vi "BMark_Get Bookmarks for VI.vi"(0 "VI":T2, 1 "App Infos In":T3[](array[typedef]), 7 "VI Cache In":T2[](array[typedef]), 9 "Bookmark Cache In":cluster{"BookmarkInfo":T1}[](array[cluster]), 11 "Error In":errorcluster, 12 "App Cache In":refnum<vi>[](array[refnum])) -> (3 "App Infos Out":T3[](array[typedef]), 4 "Bookmarks":T4, 6 "Possible Undisplayed Bookmarks":bool, 8 "VI Cache Out":T2[](array[typedef]), 10 "Bookmark Cache Out":cluster{"BookmarkInfo":T1}[](array[cluster]), 14 "App Cache Out":refnum<vi>[](array[refnum]), 15 "Error Out":errorcluster)   [LabVIEW 2018, in "Bookmark Manager.lvlib"]
uses:
  Bookmark Manager.lvlib
  Controls/BMark_VI_Identifier.ctl
  <vilib>/addons/analyzer/_analyzerctrls.llb/VIAnCtl Analysis App Info.ctl
  Controls/BMark_Array of Bookmarks.ctl
  Controls/BMark_Bookmark Cluster.ctl
  <vilib>/Utility/miscctls.llb/LVBookmarkInfoTypeDef.ctl
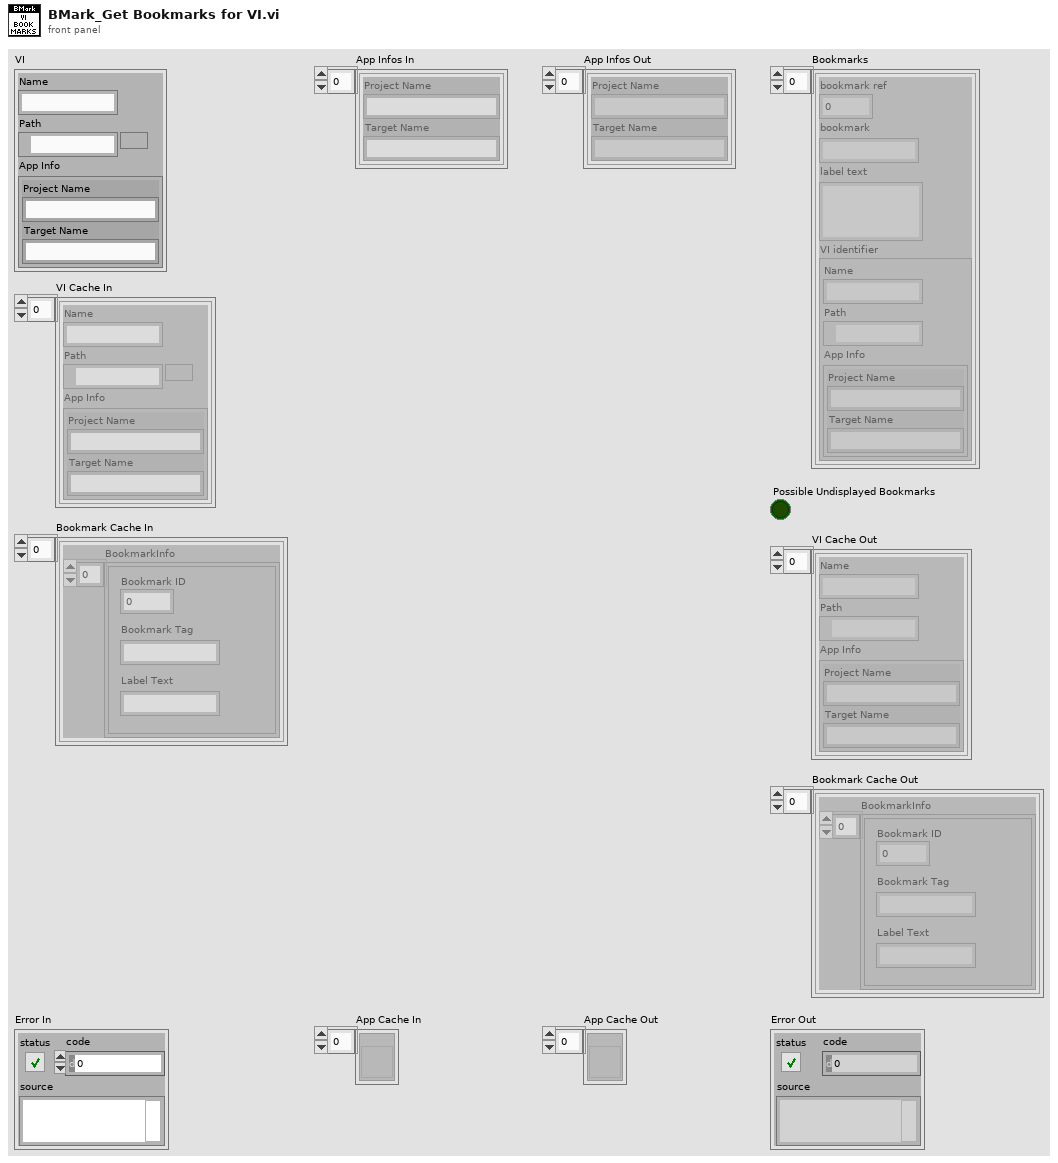
[diagram p1: front panel]
types:
  T1 = typedef "LVBookmarkInfoTypeDef.ctl" = cluster{"Bookmark ID":u32, "Bookmark Tag":string, "Label Text":string}[]
  T2 = typedef "Bookmark Manager.lvlib/BMark_VI_Identifier.ctl" = cluster{"Name":string, "Path":path, "App Info":T3}
  T3 = typedef "VIAnCtl Analysis App Info.ctl" = cluster{"Project Name":string, "Target Name":string}
  T4 = typedef "Bookmark Manager.lvlib/BMark_Array of Bookmarks.ctl" = T5[]
  T5 = typedef "Bookmark Manager.lvlib/BMark_Bookmark Cluster.ctl" = cluster{"bookmark ref":i32, "bookmark":string, "label text":string, "VI identifier":T2}
  T6 = cluster{"Bookmark Reference":u32, "Bookmark Tag":string, "Label Text":string, "VI":T2}
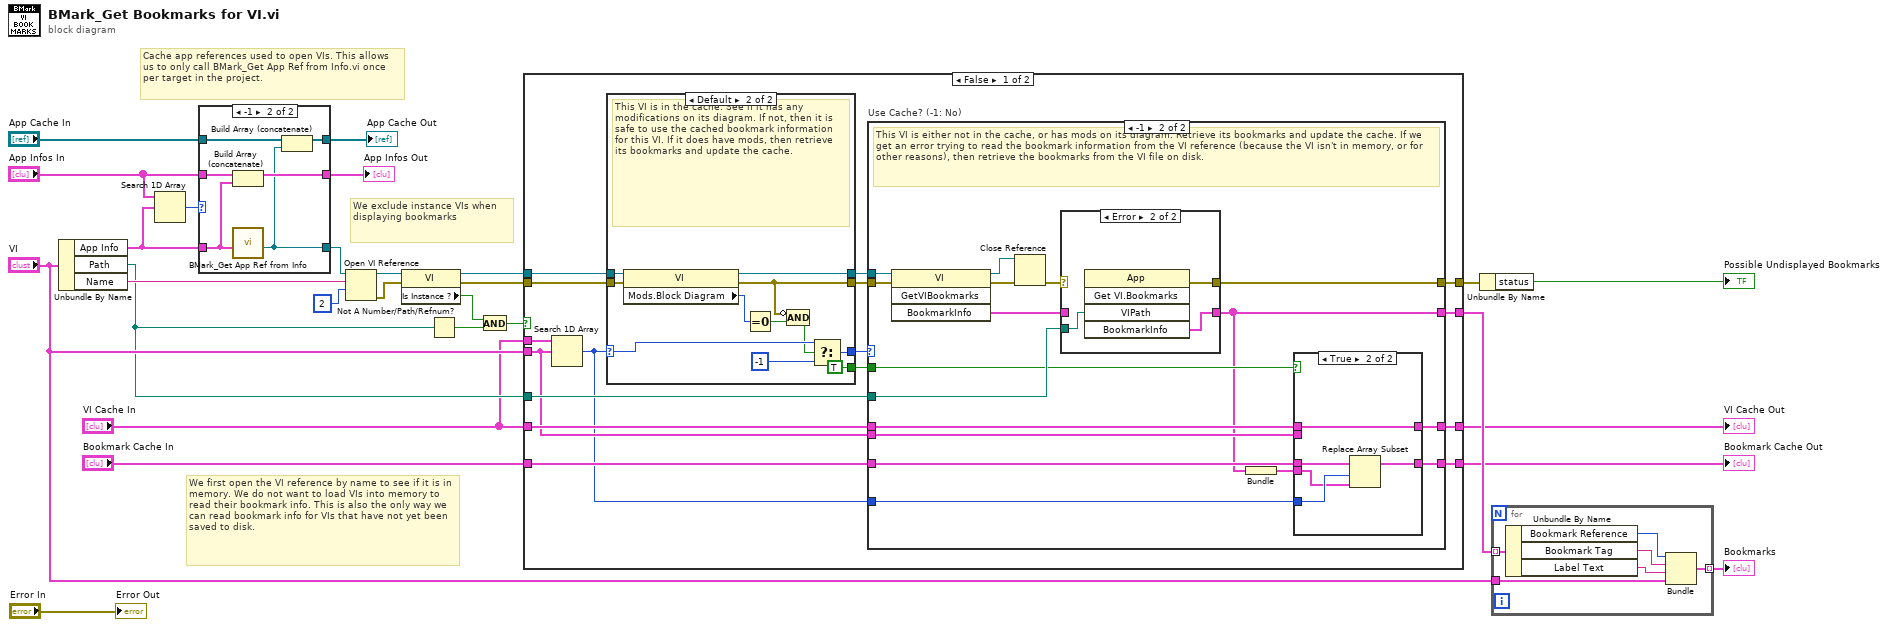
[diagram p0: block diagram]
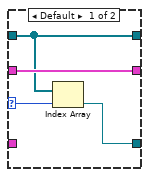
[diagram p2: hidden frame]
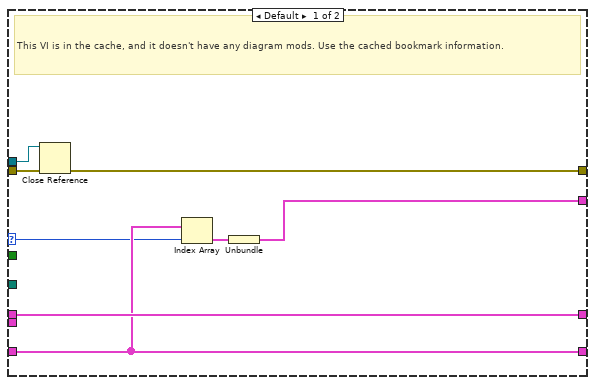
[diagram p4: hidden frame]
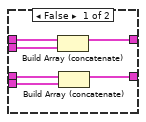
[diagram p5: hidden frame]
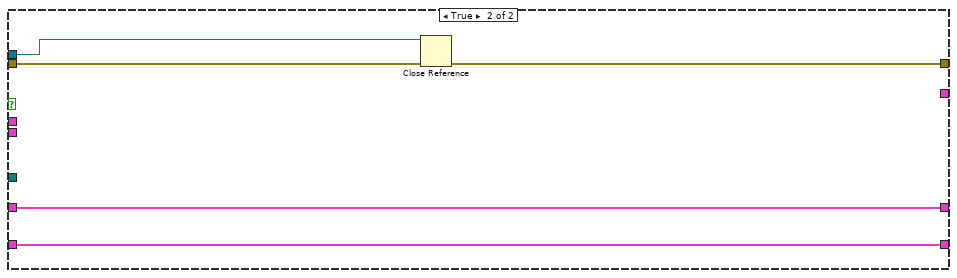
[diagram p7: hidden frame]
diagram:
  # "Cache app references used to open VIs. This allows us to only call BMark_Get App Ref from Info.vi once per target in the project."
  # "We exclude instance VIs when displaying bookmarks"
  # "We first open the VI reference by name to see if it is in memory. We do not want to load VIs into memory to read their bookmark info. This is also the only way we can read bookmark info for VIs that have not yet been saved to disk."
  n1 = Unbundle By Name("VI") -> ("App Info"=w16:T3, "Path"=w6:path, "Name"=w25:string)
  n2 = Search 1D Array(1D array="App Infos In", element=w16) -> (index of element=w15:i32)  [unwired: 1 in]
  n3 = case shown="-1" w15 {
    selector: w15 -> [w31 _]
    tunnel: [w29 w32] -> w24
    tunnel: w16 -> [_ w36]
    tunnel: "App Infos In" -> [w30 w37]
    tunnel: "App Cache In" -> [w28 w34]
    tunnel: [w28 w33] -> w12
    tunnel: [w30 w35] -> w11
    frame Default {
      n4 = Index Array(array=w28, index=w31) -> (element=w29:refnum<vi>)
    }
    frame -1 {
      n5 = Build Array (concatenate)(w37, w36) -> (w35:T3[])
      n6 = call "BMark_Get App Ref from Info.vi"("Analysis App Info"=w36) -> ("Analysis App ref"=w32:refnum<vi>)  [unwired: 9 in, 1 out]
      n7 = Build Array (concatenate)(w34, w32) -> (w33:refnum<vi>[])
    }
  }
  "App Infos Out" <- w11
  "App Cache Out" <- w12
  n8 = Open VI Reference(application reference (local)=w24, vi path=w25, options=2) -> (vi reference=w21:refnum<vi>, error out=w10:errorcluster)  [unwired: 3 in]
  n9 = property class="VI"(reference=w21, error in=w10) -> (reference out=w9:refnum<vi>, error out=w17:errorcluster, "Is Instance ?"=w20:bool)
  n10 = Not A Number/Path/Refnum?(number/path/refnum=w6) -> (NaN/Path/Refnum?=w19:bool)
  n11 = And(x=w20, y=w19) -> (x .and. y?=w18:bool)
  n12 = case shown="False" w18 {
    tunnel: w17 -> [w53 w113]
    tunnel: [w48 _] -> w7
    tunnel: w9 -> [w51 w111]
    tunnel: [w47 w112] -> w5
    tunnel: "VI" -> [w43 _]
    tunnel: "VI Cache In" -> [w49 _]
    tunnel: w6 -> [w46 _]
    tunnel: "VI Cache In" -> [w45 w110]
    tunnel: [w44 w110] -> w3
    tunnel: "Bookmark Cache In" -> [w42 w109]
    tunnel: [w41 w109] -> w1
    frame False {
      n13 = Search 1D Array(1D array=w49, element=w43) -> (index of element=w38:i32)  [unwired: 1 in]
      n14 = case shown="Default" w38 {
        selector: w38 -> [w54 w64]
        tunnel: w53 -> [w55 w67]
        tunnel: [w55 w57] -> w52
        tunnel: w51 -> [w56 w66]
        tunnel: [w56 w65] -> w50
        tunnel: [w54 w61] -> w40
        tunnel: [_ TRUE] -> w39
        frame -1 {
          # "This VI is not in the cache. We need to retrieve its bookmark information."
        }
        frame Default {
          # "This VI is in the cache. See if it has any modifications on its diagram. If not, then it is safe to use the cached bookmark information for this VI. If it does have mods, then retrieve its bookmarks and update the cache."
          n15 = property class="VI"(reference=w66, error in=w67) -> (reference out=w65:refnum<vi>, error out=w57:errorcluster, "Mods.Block Diagram"=w63:u32)
          n16 = Equal To 0?(x=w63) -> (x = 0?=w62:bool)
          n17 = Compound Arithmetic op=AND(invert w57, w62) -> (w58:bool)
          n18 = Select(t=w64, s=w58, f=-1) -> (s? t:f=w61:i32)
        }
      }
      n19 = case "Use Cache? (-1: No)" shown="-1" w40 {
        selector: w40 -> [w69 _]
        tunnel: w52 -> [w75 w92]
        tunnel: w50 -> [w74 w91]
        tunnel: [w68 w76] -> w48
        tunnel: [w73 w86] -> w47
        tunnel: w46 -> [_ w85]
        tunnel: w45 -> [w72 w84]
        tunnel: [w72 w81] -> w44
        tunnel: w43 -> [_ w83]
        tunnel: w42 -> [w71 w82]
        tunnel: [w71 w80] -> w41
        tunnel: w39 -> [_ w79]
        tunnel: w38 -> [_ w78]
        frame Default {
          # "This VI is in the cache, and it doesn't have any diagram mods. Use the cached bookmark information."
          n20 = Close Reference(reference=w74, error in (no error)=w75) -> (error out=w73:errorcluster)
          n21 = Index Array(array=w71, index=w69) -> (element=w70:cluster{"BookmarkInfo":T1})
          n22 = Unbundle(w70) -> ("BookmarkInfo"=w68:T1)
        }
        frame -1 {
          # "This VI is either not in the cache, or has mods on its diagram. Retrieve its bookmarks and update the cache. If we get an error trying to read the bookmark information from the VI reference (because the VI isn't in memory, or for other reasons), then retrieve the bookmarks from the VI file on disk."
          n23 = invoke class="VI" method="GetVIBookmarks"(reference=w91, error in=w92) -> (reference out=w90:refnum<vi>, error out=w89:errorcluster, "BookmarkInfo"=w87:T1)  [unwired: 2 in, 1 out]
          n24 = Close Reference(reference=w90, error in (no error)=w89) -> (error out=w88:errorcluster)
          n25 = case shown="Error" w88 {
            selector: w88 -> [w104 _]
            tunnel: w87 -> [w105 _]
            tunnel: [w105 w107] -> w76
            tunnel: [w104 w108] -> w86
            tunnel: w85 -> [_ w106]
            frame No Error {
            }
            frame Error {
              n26 = invoke class="App" method="Get VI.Bookmarks"("VIPath"=w106) -> (error out=w108:errorcluster, "BookmarkInfo"=w107:T1)  [unwired: 4 in, 3 out]
            }
          }
          n27 = Bundle("BookmarkInfo"=w76) -> (w77:cluster{"BookmarkInfo":T1})  [unwired: 1 in]
          n28 = case shown="True" w79 {
            tunnel: w84 -> [w98 w103]
            tunnel: w83 -> [w97 _]
            tunnel: w82 -> [w96 w102]
            tunnel: [w95 w103] -> w81
            tunnel: [w94 w101] -> w80
            tunnel: w77 -> [w93 w99]
            tunnel: w78 -> [_ w100]
            frame False {
              n29 = Build Array (concatenate)(w98, w97) -> (w95:T2[])
              n30 = Build Array (concatenate)(w96, w93) -> (w94:cluster{"BookmarkInfo":T1}[])
            }
            frame True {
              n31 = Replace Array Subset(array=w102, new element=w99, index=w100) -> (w101:cluster{"BookmarkInfo":T1}[])
            }
          }
        }
      }
    }
    frame True {
      n32 = Close Reference(reference=w111, error in (no error)=w113) -> (error out=w112:errorcluster)
    }
  }
  "VI Cache Out" <- w3
  "Bookmark Cache Out" <- w1
  n33 = Unbundle By Name(w5) -> ("status"=→"Possible Undisplayed Bookmarks":bool)
  n34 = for {
    tunnel: w7 -> [w119] mode=indexing
    tunnel: "VI" -> [w115]
    tunnel: [w118] -> w26 mode=indexing
    n35 = Unbundle By Name(w119) -> ("Bookmark Reference"=w117:u32, "Bookmark Tag"=w116:string, "Label Text"=w114:string)
    n36 = Bundle("Bookmark Reference"=w117, "Bookmark Tag"=w116, "Label Text"=w114, "VI"=w115) -> (w118:T6)  [unwired: 1 in]
  }
  "Bookmarks" <- w26
  "Error Out" <- "Error In"
